vi "Create.vi"(11 "session info":T1[](array[typedef])) -> (3 "connection map":refnum<class "Connection Map.lvclass">)   [LabVIEW 2020, in "Plug-In SDK Session Management V1 API.lvlib" / "Connection Map.lvclass"]
uses:
  Connection Map.lvclass
  gRPC/Generated APIs/ni/measurementlink/sessionmanagement/v1/RPC Messages/ni_measurementlink_sessionmanagement_v1_SessionInformation.ctl
  gRPC/Generated APIs/ni/measurementlink/sessionmanagement/v1/RPC Messages/nidevice_grpc_Session.ctl
  gRPC/Generated APIs/ni/measurementlink/sessionmanagement/v1/RPC Messages/ni_measurementlink_sessionmanagement_v1_ChannelMapping.ctl
  Connection Map.lvclass/Connection Map.ctl
  Session Reservation/Connection.ctl
  Session Reservation/Connection with Session.ctl
  <vilib>/Utility/miscctls.llb/LVMapReplaceAction.ctl
  67109d4f-8a90-48fb-848e-9eb803cf1633.vi
  6833bef1-38e8-4ffc-9b7c-737d4f73208b.vi
  1a8415d4-131e-4342-b989-234b7520ab8c.vi
  Session Reservation/Session Reservation.lvclass
  gRPC/Generated APIs/ni/measurementlink/sessionmanagement/v1/ni.measurementlink.sessionmanagement.v1.lvlib
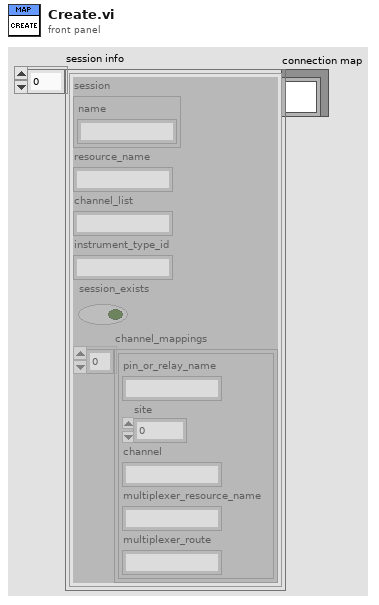
[diagram p1: front panel]
types:
  T1 = typedef "ni.measurementlink.sessionmanagement.v1.lvlib/ni_measurementlink_sessionmanagement_v1_SessionInformation.ctl" = cluster{"session":T2, "resource_name":string, "channel_list":string, "instrument_type_id":string, "session_exists":bool, "channel_mappings":T3[]}
  T2 = typedef "ni.measurementlink.sessionmanagement.v1.lvlib/nidevice_grpc_Session.ctl" = cluster{"name":string}
  T3 = typedef "ni.measurementlink.sessionmanagement.v1.lvlib/ni_measurementlink_sessionmanagement_v1_ChannelMapping.ctl" = cluster{"pin_or_relay_name":string, "site":i32, "channel":string, "multiplexer_resource_name":string, "multiplexer_route":string}
  T4 = typedef "Plug-In SDK Session Management V1 API.lvlib/Session Reservation.lvclass/Connection with Session.ctl" = cluster{"connection":T5, "session":variant}
  T5 = typedef "Plug-In SDK Session Management V1 API.lvlib/Session Reservation.lvclass/Connection.ctl" = cluster{"pin or relay name":string, "site":i32, "instrument type id":string, "channel":string}
  T6 = typedef "LVMapReplaceAction.ctl" = enum32{"Modify Entry only if found", "Add or Modify Entry", "Delete Entry"}
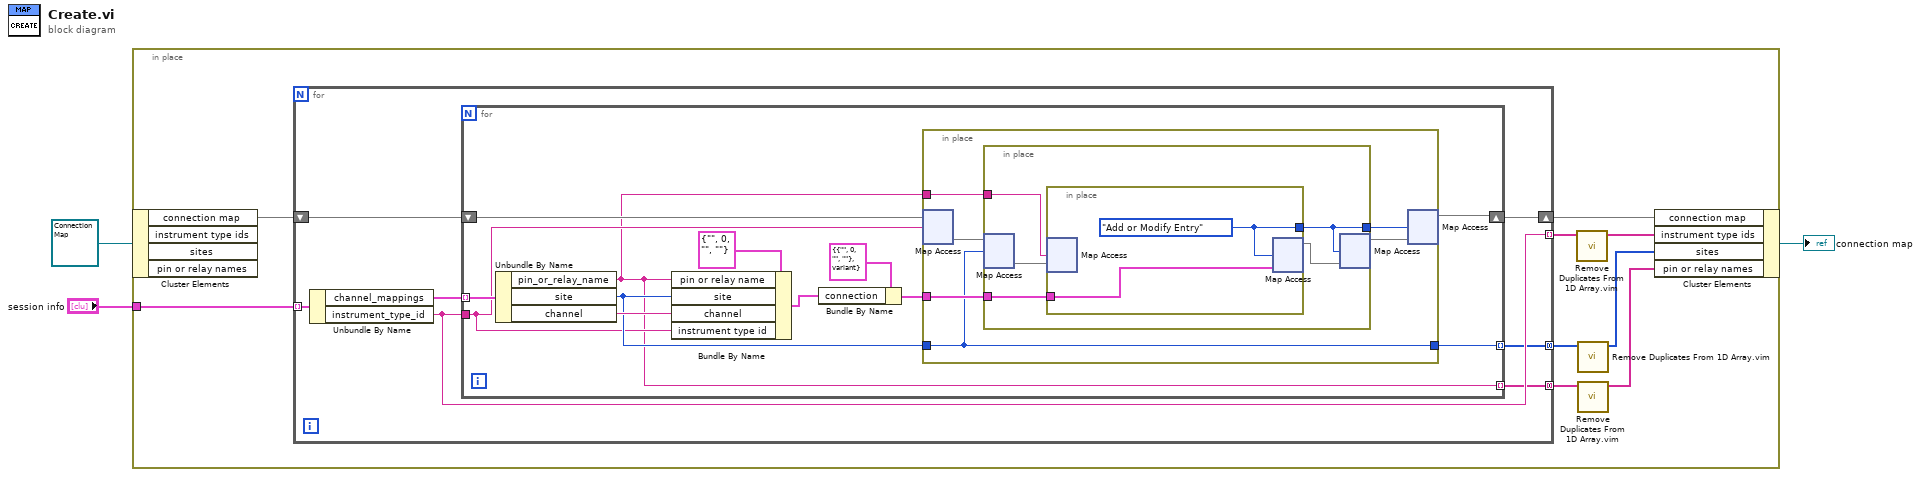
[diagram p0: block diagram]
diagram:
  n1 = in-place {
    in-place-border: "session info" -> [w12]
    n2 = in-place-cluster #1(refnum<class "Connection Map.lvclass"> refnum ("MeasurementLink Session Management.lvlib:Connection Map.lvclass")) -> ("connection map"=w11:map{string, map{i32, map{string, T4}}})  [unwired: 3 out]
    n3 = for {
      tunnel: w12 -> [w19] mode=indexing
      shift-right: [w16] -> w10
      shift-left: w11 -> [w17]
      tunnel: [w15] -> w5 mode=indexing
      tunnel: [w14] -> w9 mode=concatenating
      tunnel: [w13] -> w7 mode=concatenating
      n4 = Unbundle By Name(w19) -> ("channel_mappings"=w18:T3[], "instrument_type_id"=w15:string)
      n5 = for {
        tunnel: w18 -> [w31] mode=indexing
        tunnel: w15 -> [w23]
        shift-right: [w26] -> w16
        shift-left: w17 -> [w24]
        tunnel: [w21] -> w14 mode=indexing
        tunnel: [w20] -> w13 mode=indexing
        n6 = Unbundle By Name(w31) -> ("pin_or_relay_name"=w20:string, "site"=w25:i32, "channel"=w29:string)
        n7 = Bundle By Name(cluster=T5 {"pin or relay name"="", "site"=0, "instrument type id"="", "channel"=""} ("connection"), "pin or relay name"=w20, "site"=w25, "channel"=w29, "instrument type id"=w23) -> (w27:T5)
        n8 = Bundle By Name(cluster=T4 {"connection"={"pin or relay name"="", "site"=0, "instrument type id"="", "channel"=""}, "session"=variant} ("connection with session"), "connection"=w27) -> (w22:T4)
        n9 = in-place {
          in-place-border: w20 -> [w33]
          in-place-border: w25 -> [w32]
          in-place-border: w22 -> [w36]
          in-place-border: [w32] -> w21
          n10 = in-place-map #2(w24, w23) -> (w37:map{i32, map{string, T4}})  [unwired: 1 in, 1 out]
          n11 = in-place {
            in-place-border: w36 -> [w41]
            in-place-border: [w40] -> w35
            in-place-border: w33 -> [w38]
            n12 = in-place-map #3(w37, w32) -> (w42:map{string, T4})  [unwired: 1 in, 1 out]
            n13 = in-place {
              in-place-border: w41 -> [w44]
              in-place-border: [w43] -> w40
              w43 = LVMapReplaceAction."Add or Modify Entry" ("action")
              n14 = in-place-map #4(w42, w38) -> ()  [unwired: 1 in, 2 out]
              n15 = in-place-map #4(w44, w43) -> (w39:map{string, T4})  [unwired: 2 out]
            }
            n16 = in-place-map #3(w39, w40) -> (w34:map{i32, map{string, T4}})  [unwired: 2 out]
          }
          n17 = in-place-map #2(w34, w35) -> (w26:map{string, map{i32, map{string, T4}}})  [unwired: 2 out]
        }
      }
    }
    n18 = call "Remove Duplicates From 1D Array.vim"("array"=w5) -> ("array with duplicates removed"=w4:string[])  [unwired: 10 in]
    n19 = call "Remove Duplicates From 1D Array.vim"("array"=w9) -> ("array with duplicates removed"=w8:i32[])  [unwired: 10 in]
    n20 = call "Remove Duplicates From 1D Array.vim"("array"=w7) -> ("array with duplicates removed"=w6:string[])  [unwired: 10 in]
    n21 = in-place-cluster #1("connection map"=w10, "instrument type ids"=w4, "sites"=w8, "pin or relay names"=w6) -> (→"connection map":refnum<class "Connection Map.lvclass">)
  }
